vi "Gyro-free PID Fwd C4 Assisted Dis - Left Edge.vi"(5 "Target reflection":sgl=32.0, 7 "Threshold to Stop":i32=600, 8 "Threshold to slow":i32=400, 9 "Min. speed":i32=20, 10 "Max. speed":i32=40, 11 "EV3 in":T1) -> (3 "EV3 out":T1)   [LabVIEW 2016]
uses:
  <vilib>/NXT/Subs/LVHSConnector.ctl
  <vilib>/NXT/LegoClasses/BrickReference/BrickReference.lvclass
  <vilib>/NXT/Block Support/NXT_OutputPort.ctl
  <vilib>/NXT/Block Support/NXT_InputPort.ctl
  <vilib>/NXT/NXTIO Xnodes/NXTIONodeSubVIs/LEGOResetMotors.vi
  <vilib>/NXT/Dual Mode Library/Motors/Rotation.vi
  <vilib>/NXT/NXTIO Xnodes/NXTIONodeSubVIs/NXTMotorSteeringOn.vi
  <vilib>/NXT/NXTIO Xnodes/NXTIONodeSubVIs/NXTStopMotors.vi
  <vilib>/NXT/Dual Mode Library/Waits/Wait_Num.vi
  <vilib>/NXT/NXTIO Xnodes/NXTIOXNode/NXTIO.xnode
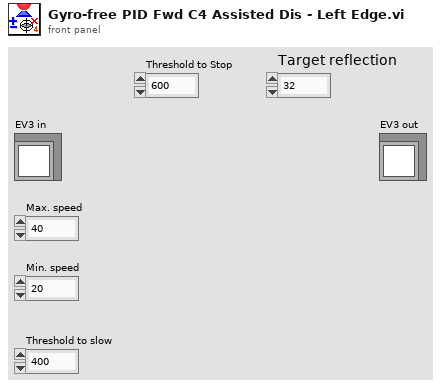
[diagram p1: front panel]
types:
  T1 = typedef "LVHSConnector.ctl" = refnum<class "BrickReference.lvclass">
  T2 = typedef "NXT_OutputPort.ctl" = u8
  T3 = typedef "NXT_InputPort.ctl" = u32
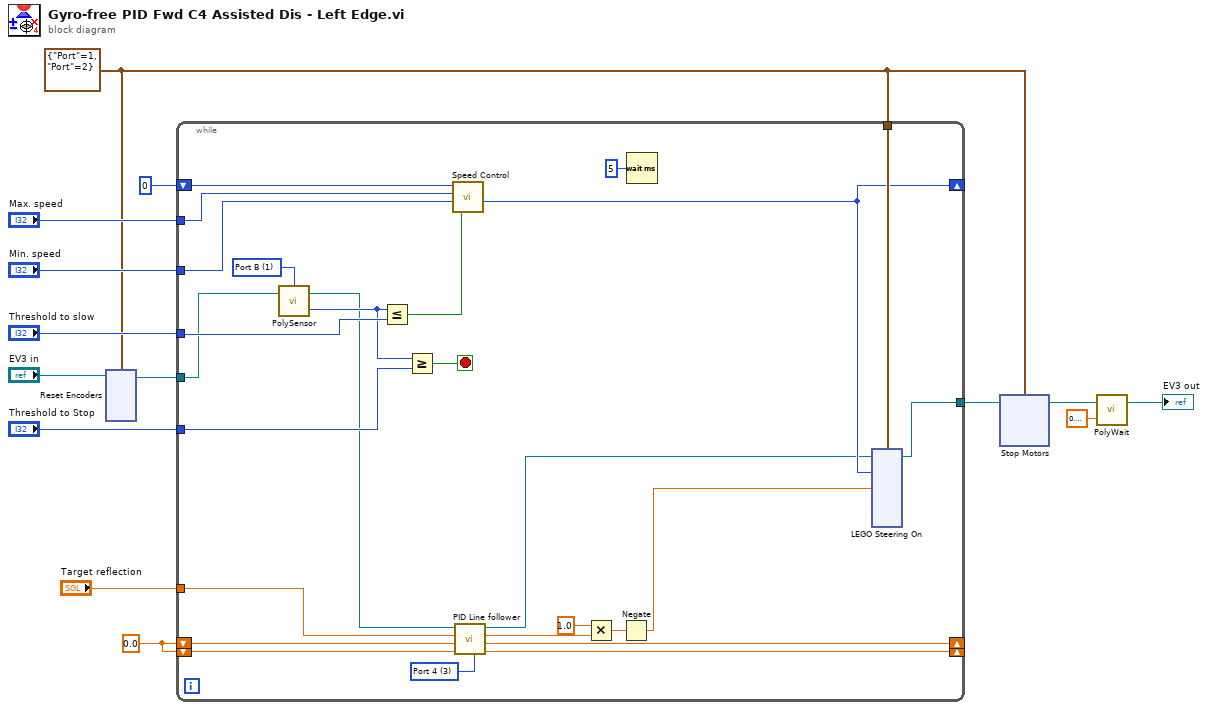
[diagram p0: block diagram]
diagram:
  w6 = cluster{"Port":T2, "Port":T2} {"Port"=1, "Port"=2} ("Motor")
  w2 = sgl 0.0
  n1 = xnode "Reset Encoders"("Motors"=w6, "NXT/EV3"="EV3 in") -> ("NXT/EV3"=w12:T1)
  n2 = while {
    tunnel: w12 -> [w32]
    tunnel: [w38] -> w8
    tunnel: w6 -> [w40]
    shift-right: [w28] -> _
    shift-left: 0 -> [w36]
    tunnel: "Min. speed" -> [w33]
    tunnel: "Max. speed" -> [w35]
    tunnel: "Threshold to slow" -> [w34]
    tunnel: "Threshold to Stop" -> [w29]
    shift-right: [w24] -> _
    shift-left: w2 -> [w27]
    shift-right: [w25] -> _
    shift-left: w2 -> [w26]
    tunnel: "Target reflection" -> [w22]
    stop <- w17 stop-if-true
    w18 = T3 3 items=["Port 1", "Port 2", "Port 3", "Port 4"] ("Port (Port 1)")
    w39 = T2 1 items=["Port A", "Port B", "Port C", "Port D"] ("Port (Port A)")
    n3 = call-poly <vilib>:"PolySensor.vi"("NXT/EV3"=w32, "Port (Port A)"=w39) -> ("Angle of Rotation"=w30:i32, "NXT/EV3"=w21:T1)  [unwired: 1 in]
    n4 = Less Or Equal?(x=w30, y=w34) -> (x <= y?=w31:bool)
    n5 = Greater Or Equal?(x=w30, y=w29) -> (x >= y?=w17:bool)
    n6 = call "Speed Control.vi"("Speed Up or Down?"=w31, "Min. speed"=w33, "Max. speed"=w35, "Ini. speed"=w36) -> ("Speed out"=w28:i32)  [unwired: 7 in]
    n7 = call "PID Line follower.vi"("Port (Port 1)"=w18, "Old Error"=w27, "Previous integral"=w26, "Target reflection"=w22, "EV3 in"=w21) -> ("New Error"=w24:sgl, "New integral"=w25:sgl, "Total error"=w23:sgl, "EV3 out"=w15:T1)  [unwired: 3 in]
    n8 = Multiply(x=sgl 1.0, y=w23) -> (x*y=w20:sgl)
    n9 = Negate(x=w20) -> (-x=w16:sgl)
    n10 = Wait (ms)(milliseconds to wait=u32 5) -> ()  [unwired: 1 out]
    n11 = xnode "LEGO Steering On"("Steering 1"=w16, "Power 1"=w28, "Motors"=w40, "NXT/EV3"=w15) -> ("NXT/EV3"=w38:T1)
  }
  n12 = xnode "Stop Motors"("Motors"=w6, "NXT/EV3"=w8) -> ("NXT/EV3"=w7:T1)
  n13 = call-poly <vilib>:"PolyWait.vi"("Time (1 sec)"=sgl 0.2, "NXT/EV3"=w7) -> ("NXT/EV3"=→"EV3 out":T1)  [unwired: 2 in]
